vi "set array to zero (dbl 2d).vi"(1 "array in":dbl[][](array[numeric])) -> (0 "array out":dbl[][](array[numeric]))   [LabVIEW 2012, in "common.lvlib"]
uses:
  common.lvlib
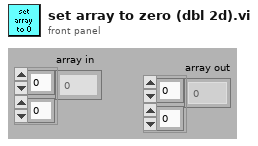
[diagram p1: front panel]
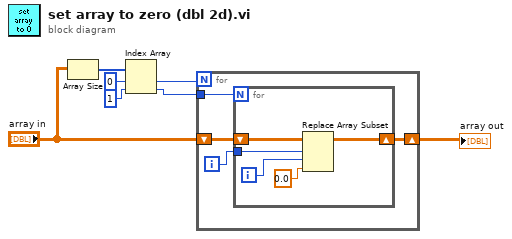
[diagram p0: block diagram]
diagram:
  n1 = Array Size(array="array in") -> (size(s)=w6:i32[])
  n2 = Index Array(array=w6, index #1=0 ("index"), index #2=1 ("index")) -> (element #1=w3:i32, element #2=w2:i32)
  n3 = for {
    N: w3 -> [_]
    tunnel: w2 -> [w10]
    shift-right: [w8] -> w1
    shift-left: "array in" -> [w11]
    i -> [w9]
    n4 = for {
      N: w10 -> [_]
      shift-right: [w12] -> w8
      shift-left: w11 -> [w16]
      tunnel: w9 -> [w15]
      i -> [w14]
      n5 = Replace Array Subset(array=w16, new element=0.0 ("new element/subarray"), index (row)=w15, index (col)=w14) -> (w12:dbl[][])
    }
  }
  "array out" <- w1
